vi "Perform Step.vi"(8 "error in (no error)":errorcluster, 11 "Keyboard Macro in":refnum<class "Keyboard Macro.lvclass">) -> (0 "error out":errorcluster, 2 "Result":T1, 3 "Keyboard Macro out":refnum<class "Keyboard Macro.lvclass">)   [LabVIEW 2023, in "MacroAssert.lvlib" / "Keyboard Macro.lvclass"]
uses:
  Keyboard Macro.lvclass
  Keyboard Macro.lvclass/Keyboard Macro.ctl
  MacroAssert.lvlib
  CTLs/Report Data.ctl
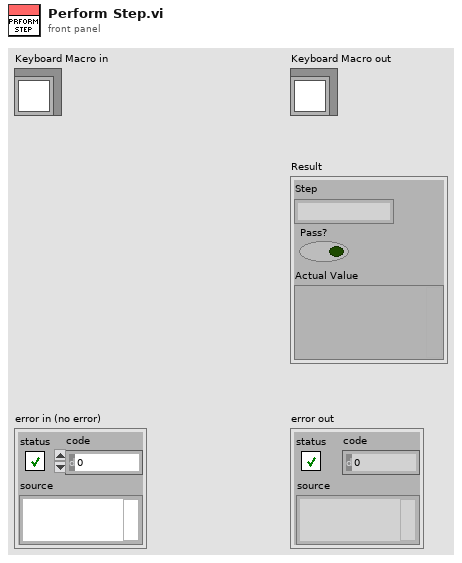
[diagram p1: front panel]
types:
  T1 = typedef "MacroAssert.lvlib/Report Data.ctl" = cluster{"Step":string, "Pass?":bool, "Actual Value":variant}
  T2 = typedef "MacroAssert.lvlib/Step Type V3.ctl" = enum16{"Mouse Move", "Mouse Click", "Key Press", "Wait", "Mouse Down", "Mouse Up", "Key Down", "Key Up", "Test Assertion", "Maximize Window", "Restore Window", "Minimize Window", "Close Window", "Bring Window to Front", "Send Window to Back"}
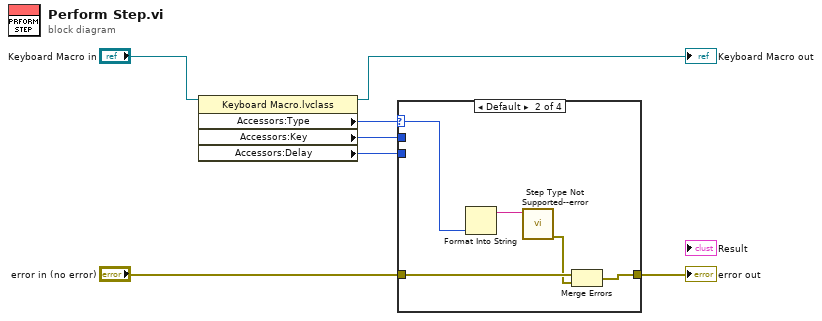
[diagram p0: block diagram]
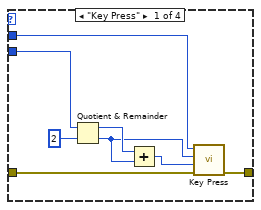
[diagram p2: hidden frame]
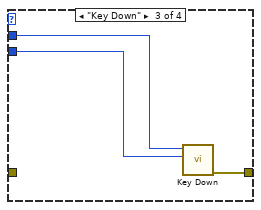
[diagram p3: hidden frame]
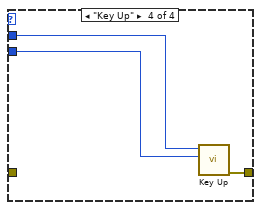
[diagram p4: hidden frame]
diagram:
  n1 = property class="Keyboard Macro.lvclass"(reference="Keyboard Macro in") -> (reference out=→"Keyboard Macro out":refnum<class "Keyboard Macro.lvclass">, "Accessors:Type"=w4:T2, "Accessors:Key"=w2:u8, "Accessors:Delay"=w1:i32)  [unwired: 1 in, 1 out]
  n2 = case shown="Default" w4 {
    selector: w4 -> [_ w20 _ _]
    tunnel: w1 -> [w14 _ w22 w25]
    tunnel: w2 -> [w9 _ w21 w24]
    tunnel: [w15 w16 w23 w26] -> w3
    tunnel: "error in (no error)" -> [w8 w18 _ _]
    frame "Key Press" {
      n3 = Quotient & Remainder(x=w14, y=2) -> (x-y*floor(x/y)=w12:i32, floor(x/y)=w10:i32)
      n4 = Add(x=w12, y=w10) -> (x+y=w11:i32)
      n5 = call "Key Press.vi"("error in (no error)"=w8, "ms wait after up (20)"=w11, "ms wait after down (80)"=w10, "Virtual Key"=w9) -> ("error out"=w15:errorcluster)  [unwired: 7 in]
    }
    frame Default {
      n6 = Format Into String(w20) -> (resulting string=w19:string)  [unwired: 3 in, 1 out]
      n7 = call "Step Type Not Supported--error.vi"("Step Type"=w19) -> ("error out"=w17:errorcluster)  [unwired: 10 in]
      n8 = Merge Errors(w18, w17) -> (w16:errorcluster)
    }
    frame "Key Down" {
      n9 = call "Key Down.vi"("delay in ms (80)"=w22, "Virtual Key"=w21) -> ("error out"=w23:errorcluster)  [unwired: 9 in]
    }
    frame "Key Up" {
      n10 = call "Key Up.vi"("delay in ms (20)"=w25, "Virtual Key"=w24) -> ("error out"=w26:errorcluster)  [unwired: 9 in]
    }
  }
  "error out" <- w3
